vi "Post Process Ctl Index.vi"(8 "Call Procedure?":bool, 11 "Ctl Index in":u8) -> (0 "Exit?":bool, 3 "Ctl Index out":u8)   [LabVIEW 2014, in "hse-db.lvlib" / "MySQL (TCP).lvlib"]
uses:
  MySQL (TCP).lvlib
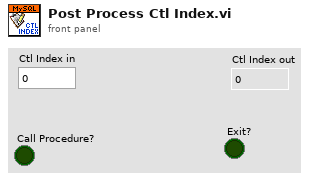
[diagram p1: front panel]
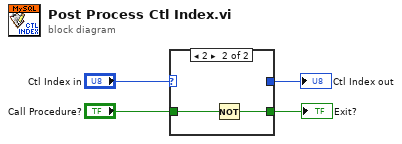
[diagram p0: block diagram]
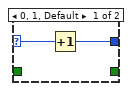
[diagram p2: hidden frame]
diagram:
  n1 = case shown="2" "Ctl Index in" {
    selector: "Ctl Index in" -> [w6 _]
    tunnel: "Call Procedure?" -> [_ w8]
    tunnel: [_ w7] -> w4
    tunnel: [w5 _] -> w1
    frame 0, 1, Default {
      n2 = Increment(x=w6) -> (x+1=w5:u8)
    }
    frame 2 {
      n3 = Not(x=w8) -> (.not. x?=w7:bool)
    }
  }
  "Exit?" <- w4
  "Ctl Index out" <- w1
